vi "Express VI - Dual Channel Spectral Measurement.vi"() -> ()   [LabVIEW 2023]
doc: "This example demonstrates how to use the Dual Channel Spectral Measurement Express VI to analyze the frequency response of a bandpass digital filter by comparing the input signal (Pre-Filtered) to the output signal (Filtered). This example also demonstrates how to compare the frequency response to arbitrary specifications to determine whether the digital filter meets your requirements. Various filter design parameters, such as topology and order, changed from the block diagram to successfully design the filter. This example uses a white noise signal as the stimulus of the filter, measures the frequency response between this stimulus and the response of the filter, and then tests if the result falls within some arbitrary limits."
panel:
  out "Passed":bool=TRUE
  out "Waveform Graph":dynamicdata(graph)
  in  "Stop":bool
  in  "Filter Upper Cut-Off":i32(slide)=3800 scale=0.0..8000.0
  in  "Filter Lower Cut-Off":i32(slide)=2200 scale=0.0..8000.0
  # "Overview: Demonstrates how to use the Dual Channel Spectral Measurement Express VI to analyze the frequency response of a bandpass digital filter by comparing the input signal (before the filter) to the output signal (after the filter)\nRequirements: LabVIEW Full Development System\nInstructions:\n1. Run the VI.\n2. See the Filter response along with the Upper and Lower Limits (set by Mask and Limit Testing Express VI) and see whether the calculated Filter response is within the specifications. \n3. You can change the Filter Lower Cut-Off and Filter Upper Cut-Off frequencies.\n4. Click Stop to stop the VI."
  # "The LED above indicates whether or not the frequency response of the bandpass digital filter is within the limits specified in the Properties of the Mask and Limit Testing Express VI."
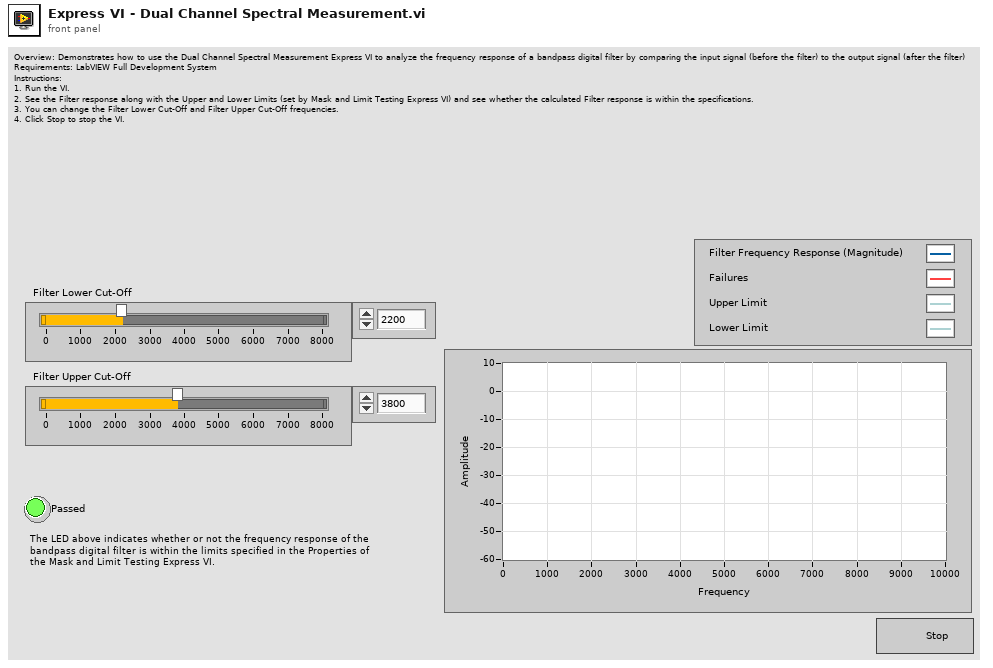
[diagram p1: front panel]
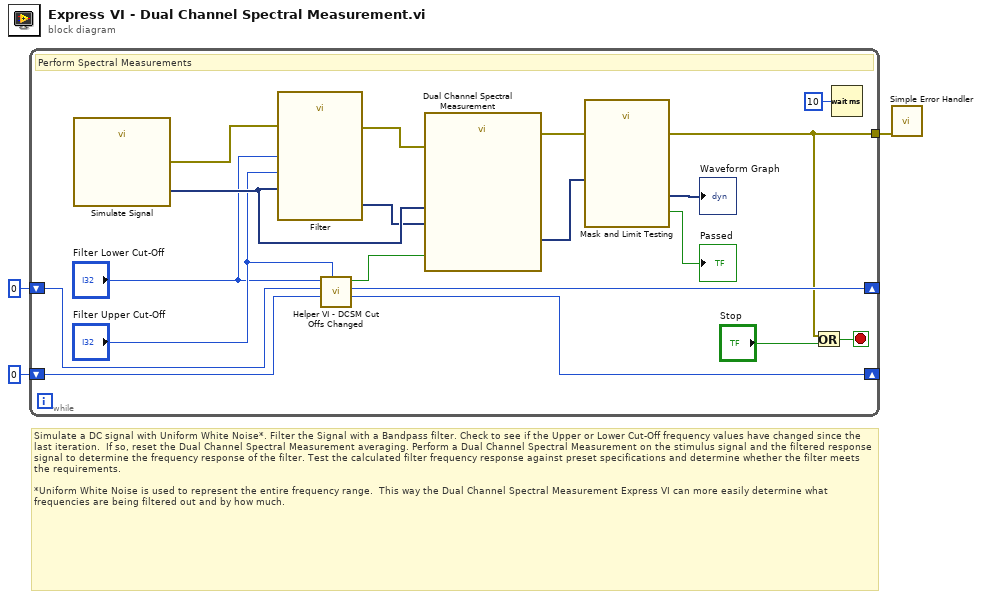
[diagram p0: block diagram]
diagram:
  # "Simulate a DC signal with Uniform White Noise*. Filter the Signal with a Bandpass filter. Check to see if the Upper or Lower Cut-Off frequency values have changed since the last iteration.  If so, reset the Dual Channel Spectral Measurement averaging. Perform a Dual Channel Spectral Measurement on the stimulus signal and the filtered response signal to determine the frequency response of the filter. Test the calculated filter frequency response against preset specifications and determine whether the filter meets the requirements.\n\n*Uniform White Noise is used to represent the entire frequency range.  This way the Dual Channel Spectral Measurement Express VI can more easily determine what frequencies are being filtered out and by how much."
  n1 = while {
    shift-right: [w7] -> _
    shift-left: 0 ("New Upper Cut-Off out") -> [w9]
    shift-right: [w6] -> _
    shift-left: 0 ("New Lower Cut-Off out") -> [w8]
    tunnel: [w4] -> w1
    stop <- w5 stop-if-true
    # "Perform Spectral Measurements"
    n2 = call "Simulate Signal"() -> ("Simulated Signal"=w15:dynamicdata, "error out"=w16:errorcluster)  [unwired: 14 in]
    n3 = call "Filter"("error in (no error)"=w16, "Lower Cut-Off"="Filter Lower Cut-Off", "Upper Cut-Off"="Filter Upper Cut-Off", "Signal"=w15) -> ("error out"=w17:errorcluster, "Filtered Signal"=w14:dynamicdata)  [unwired: 6 in]
    n4 = call "Helper VI - DCSM Cut Offs Changed.vi"("New Upper Cut-Off"="Filter Upper Cut-Off", "Old Lower Cut-Off"=w8, "Old Upper Cut-Off"=w9, "New Lower Cut-Off"="Filter Lower Cut-Off") -> ("New Lower Cut-Off out"=w6:i32, "New Upper Cut-Off out"=w7:i32, "Changed?"=w19:bool)  [unwired: 5 in]
    n5 = call "Dual Channel Spectral Measurement"("error in (no error)"=w17, "Restart Averaging (F)"=w19, "Input Signal B"=w14, "Input Signal A"=w15) -> ("error out"=w18:errorcluster, "Magnitude"=w22:dynamicdata)  [unwired: 5 in, 1 out]
    n6 = call "Mask and Limit Testing"("error in"=w18, "Signals"=w22) -> ("error out"=w4:errorcluster, "Passed"=→"Passed":bool, "Tested Signals"=→"Waveform Graph":dynamicdata)  [unwired: 6 in, 1 out]
    n7 = Or(x=w4, y="Stop") -> (x .or. y?=w5:bool)
    n8 = Wait (ms)(milliseconds to wait=u32 10) -> ()  [unwired: 1 out]
  }
  n9 = call <vilib>:"Simple Error Handler.vi"("error in (no error)"=w1) -> ()  [unwired: 4 in, 5 out]
